vi "Lockin.DAQ.Start.AO.vi"(8 "error in (no error)":errorcluster, 11 "Lockin.DAQ in":refnum<class "Instrument.DAQ.lvclass">) -> (0 "error out":errorcluster, 3 "Lockin.DAQ out":refnum<class "Instrument.DAQ.lvclass">)   [LabVIEW 2019, in "Instrument.DAQ.lvclass"]
uses:
  Instrument.DAQ.lvclass
  Instrument.DAQ.lvclass/Instrument.DAQ.ctl
  <vilib>/DAQmx/write.llb/DAQmx Write (Analog 1D Wfm NChan NSamp).vi
  <vilib>/DAQmx/miscellaneous.llb/DAQmx Fill In Error Info.vi
panel:
  out "reset indicator":bool
  out "Array":u32[](array[numeric])
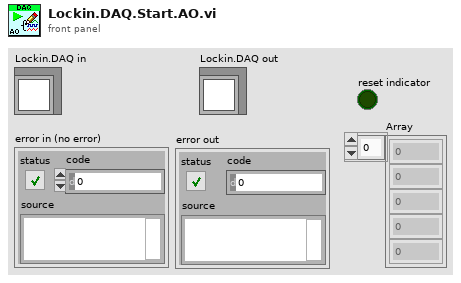
[diagram p1: front panel]
types:
  T1 = typedef "Instrument.DAQ.lvclass/DAQType-enum.ctl" = enum16{"None", "USB 4431", "PXI 446x"}
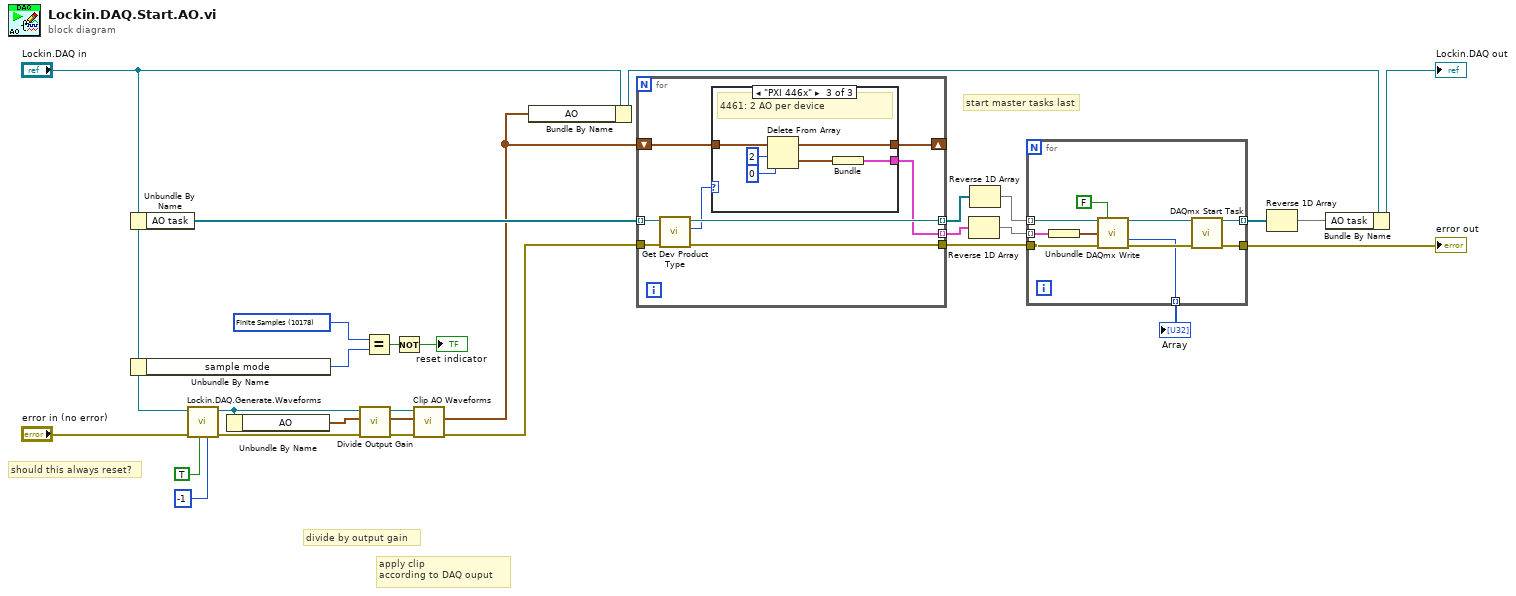
[diagram p0: block diagram]
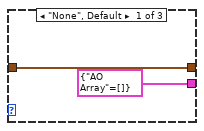
[diagram p2: hidden frame]
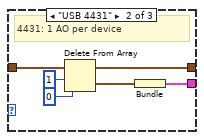
[diagram p3: hidden frame]
diagram:
  w15 = 10178 items=["Finite Samples"=10178, "Continuous Samples"=10123] ("sample mode 2")
  # "start master tasks last"
  # "apply clip\naccording to DAQ ouput"
  # "divide by output gain"
  # "should this always reset?"
  n1 = Unbundle By Name("Lockin.DAQ in") -> ("AO task"=w24:refnum<k21>[])
  n2 = Unbundle By Name("Lockin.DAQ in") -> ("sample mode"=w14:i32)
  n3 = call "Lockin.DAQ.Generate.Waveforms.vi"("sweep index"=-1, "Reset Phase?"=TRUE ("reset signal"), "error in (no error)"="error in (no error)", "Lockin.DAQ"="Lockin.DAQ in") -> ("error out"=w10:errorcluster, "Lockin.DAQ"=w5:refnum<class "Instrument.DAQ.lvclass">)  [unwired: 6 in]
  n4 = Unbundle By Name(w5) -> ("AO"=w4:waveform(dbl)[])
  n5 = call "Divide Output Gain.vi"("error in (no error)"=w10, "WFM in"=w4, "Lockin.DAQ"=w5) -> ("error out"=w11:errorcluster, "WFM out"=w13:waveform(dbl)[], "Lockin.DAQ out"=w12:refnum<class "Instrument.DAQ.lvclass">)  [unwired: 6 in]
  n6 = Equal?(x=w15, y=w14) -> (x = y?=w28:bool)
  n7 = Not(x=w28) -> (.not. x?=→"reset indicator":bool)
  n8 = call "Clip AO Waveforms.vi"("error in (no error)"=w11, "AO []"=w13, "Lockin.DAQ in"=w12) -> ("error out"=w9:errorcluster, "Clipped AO []"=w1:waveform(dbl)[])  [unwired: 6 in, 1 out]
  n9 = Bundle By Name(cluster="Lockin.DAQ in", "AO"=w1) -> (w2:refnum<class "Instrument.DAQ.lvclass">)
  n10 = for {
    tunnel: w24 -> [w36] mode=indexing
    shift-right: [w34] -> _
    shift-left: w1 -> [w35]
    tunnel: [w29] -> w23 mode=indexing
    tunnel: [w33] -> w22 mode=indexing
    tunnel: w9 -> [w32]
    tunnel: [w31] -> w21
    n11 = call "Get Dev Product Type.vi"("error in (no error)"=w32, "Refnum in"=w36) -> ("error out"=w31:errorcluster, "DAQ Type"=w30:T1, "Refnum out"=w33:refnum<k21>)  [unwired: 6 in, 1 out]
    n12 = case shown="\"PXI 446x\"" w30 {
      tunnel: w35 -> [w38 w44 w50]
      tunnel: [w38 w43 w49] -> w34
      tunnel: [cluster{"AO Array":waveform(dbl)[]} {"AO Array"=[]} w41 w46] -> w29
      frame "None", Default {
      }
      frame "USB 4431" {
        # "4431: 1 AO per device"
        n13 = Delete From Array(array=w44, length=1, index=0) -> (deleted portion=w40:waveform(dbl)[], array with subset deleted=w43:waveform(dbl)[])
        n14 = Bundle("Clipped AO []"=w40) -> (w41:cluster{"Clipped AO []":waveform(dbl)[]})  [unwired: 1 in]
      }
      frame "PXI 446x" {
        # "4461: 2 AO per device"
        n15 = Delete From Array(array=w50, length=2, index=0) -> (deleted portion=w47:waveform(dbl)[], array with subset deleted=w49:waveform(dbl)[])
        n16 = Bundle("Clipped AO []"=w47) -> (w46:cluster{"Clipped AO []":waveform(dbl)[]})  [unwired: 1 in]
      }
    }
  }
  n17 = Reverse 1D Array(array=w23) -> (reversed array=w7:cluster{"Clipped AO []":waveform(dbl)[]}[])
  n18 = Reverse 1D Array(array=w22) -> (reversed array=w8:refnum<k21>[])
  n19 = for {
    tunnel: w8 -> [w52] mode=indexing
    tunnel: w21 -> [w58]
    tunnel: [w57] -> w25
    tunnel: [w56] -> w26 mode=indexing
    tunnel: w7 -> [w55] mode=indexing
    tunnel: [w53] -> w20 mode=indexing
    n20 = Unbundle(w55) -> ("Clipped AO []"=w51:waveform(dbl)[])
    n21 = call-poly <vilib>:"DAQmx Write.vi"("task/channels in"=w52, "auto start"=FALSE, "data"=w51, "error in"=w58) -> ("task out"=w59:refnum<k21>, "number of samples written per channel"=w53:u32, "error out"=w60:errorcluster)  [unwired: 9 in]
    n22 = call <vilib>:"DAQmx Start Task.vi"("task/channels in"=w59, "error in"=w60) -> ("task out"=w56:refnum<k21>, "error out"=w57:errorcluster)  [unwired: 12 in]
  }
  "error out" <- w25
  "Array" <- w20
  n23 = Reverse 1D Array(array=w26) -> (reversed array=w6:refnum<k21>[])
  n24 = Bundle By Name(cluster=w2, "AO task"=w6) -> (→"Lockin.DAQ out":refnum<class "Instrument.DAQ.lvclass">)
